vi "Read Curve Parameters.vi"(8 "error in (no error)":errorcluster, 11 "EdgeDetectionProcessor in":refnum<class "EdgeDetectionProcessor.lvclass">) -> (0 "error out":errorcluster, 2 "Curve Parameters":T1={"Extraction Mode"=0, "Edge Threshold"=75, "Edge Filter Size"=1, "Min Length"=25, "Row Search Step Size"=15, "Col Search Step Size"=15, "Max Endpoint Gap"=10, "Closed"=FALSE, "Subpixel"=FALSE} {"Max Endpoint Gap" min=0; "Col Search Step Size" min=1 max=255 step=1; "Row Search Step Size" min=1 max=255 step=1; "Min Length" min=0; "Edge Filter Size" items=["Fine", "Normal", "Controur Tracing"]; "Edge Threshold" min=1 max=65535 step=1; "Extraction Mode" items=["Normal", "Uniform Regions"]}, 3 "EdgeDetectionProcessor out":refnum<class "EdgeDetectionProcessor.lvclass">)   [LabVIEW 2018, in "EdgeDetectionProcessor.lvclass"]
uses:
  EdgeDetectionProcessor.lvclass
  <vilib>/vision/Pattern Matching.llb/IMAQ Curve Parameters.ctl
  EdgeDetectionProcessor.lvclass/EdgeDetectionProcessor.ctl
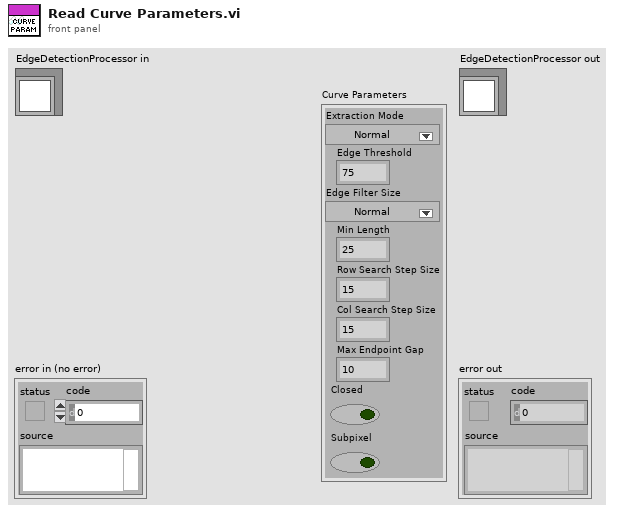
[diagram p1: front panel]
types:
  T1 = typedef "IMAQ Curve Parameters.ctl" = cluster{"Extraction Mode":u32, "Edge Threshold":i32, "Edge Filter Size":u32, "Min Length":i32, "Row Search Step Size":i32, "Col Search Step Size":i32, "Max Endpoint Gap":i32, "Closed":bool, "Subpixel":bool}
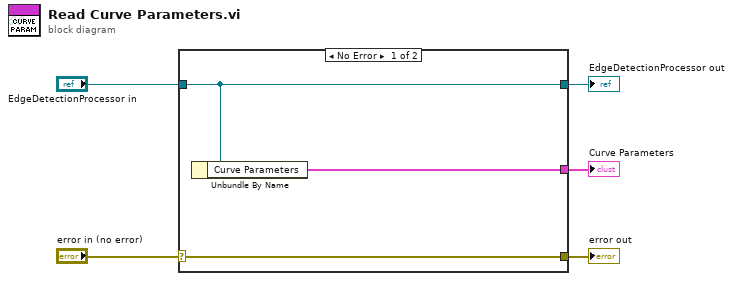
[diagram p0: block diagram]
diagram:
  n1 = case shown="No Error" "error in (no error)" {
    selector: "error in (no error)" -> [w8 w9]
    tunnel: [w8 w9] -> w4
    tunnel: [w7 w10] -> w2
    tunnel: "EdgeDetectionProcessor in" -> [w7 w10]
    tunnel: [w6 _] -> w1
    frame No Error {
      n2 = Unbundle By Name(w7) -> ("Curve Parameters"=w6:T1)
    }
    frame Error {
    }
  }
  "error out" <- w4
  "EdgeDetectionProcessor out" <- w2
  "Curve Parameters" <- w1
